vi "DAQmx Create Channel (TEDS-AI-Force-IEPE Sensor).vi"(0 "task in":refnum<k21>, 1 "maximum value":dbl=2000.0 format="%0.2f", 2 "minimum value":dbl=-2000.0 format="%0.2f", 3 "input terminal configuration":i32(ring)=-1 items=["default"=-1, "RSE"=10083, "NRSE"=10078, "Differential"=10106, "Pseudodifferential"=12529], 5 "physical channels":tag, 6 "current excitation source":i32(ring)=10200 items=["Internal"=10200, "External"=10167, "None"=10230], 7 "name to assign":string, 8 "current excitation value":dbl=0.001, 9 "units":i32(ring)=15875 items=["Newtons"=15875, "Pounds"=15876, "From Custom Scale"=10065], 11 "error in":errorcluster, 12 "custom scale name":tag) -> (4 "task out":refnum<k21>, 15 "error out":errorcluster)   [LabVIEW 2018]
doc: "Creates channel(s) that use an IEPE force sensor to measure force or load. You must configure the physical channel(s) with TEDS information to use this VI."
uses:
  nilvaiu.dll
panel:
  # "input limits"
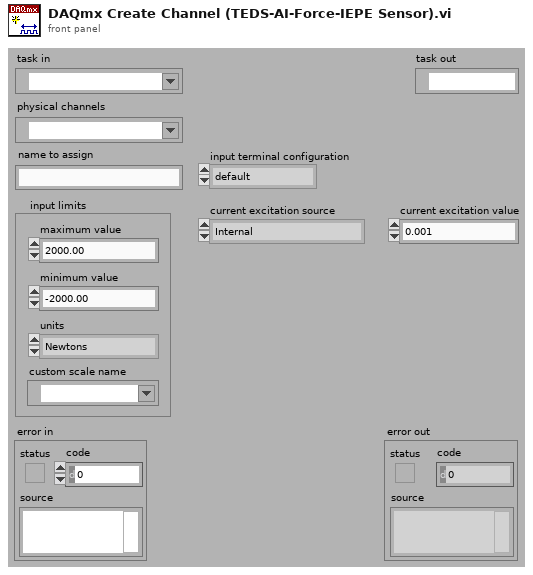
[diagram p1: front panel]
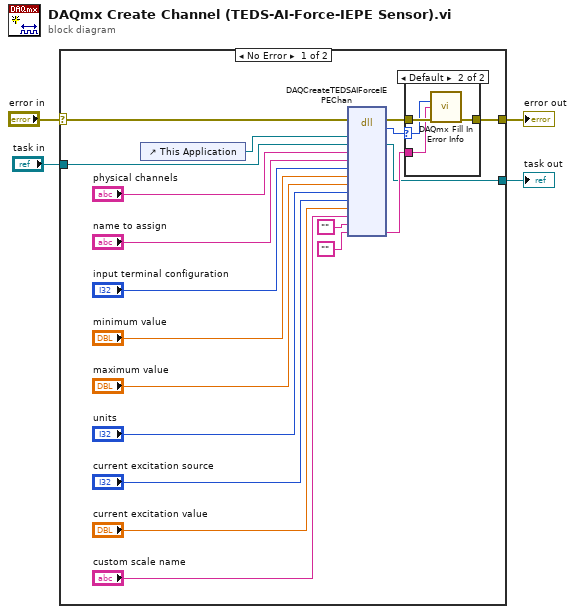
[diagram p0: block diagram]
diagram:
  n1 = case shown="No Error" "error in" {
    selector: "error in" -> [w18 w30]
    tunnel: [w17 w30] -> w2
    tunnel: "task in" -> [w16 w29]
    tunnel: [w15 w29] -> w1
    frame No Error {
      n2 = control-ref of="This Application"() -> (w20:refnum<vi>)
      n3 = dll-call lib="nilvaiu.*" fn="DAQCreateTEDSAIForceIEPEChan"(error in=w18, "lvAppRef"=w20, "refObjPtr"=w16, "physicalChannelName"="physical channels", "channelNameIn"="name to assign", "terminalConfig"="input terminal configuration", "minVal"="minimum value", "maxVal"="maximum value", "units"="units", "currentExcitSrc"="current excitation source", "excitVal"="current excitation value", "customScaleName"="custom scale name", "channelNamesOut"="", "extendedErrorInfo"="") -> (error out=w23:errorcluster, "return type"=w22:i32, "refObjPtr"=w15:refnum<k21>, "extendedErrorInfo"=w21:string)  [unwired: 13 in, 1 out]
      n4 = case shown="Default" w22 {
        selector: w22 -> [_ w26]
        tunnel: w23 -> [w24 w28]
        tunnel: [w24 w27] -> w17
        tunnel: w21 -> [_ w25]
        frame 0 {
        }
        frame Default {
          n5 = call "DAQmx Fill In Error Info.vi"("status code"=w26, "extended error info"=w25, "error in"=w28) -> ("error out"=w27:errorcluster)  [unwired: 1 in, 11 out]
        }
      }
    }
    frame Error {
    }
  }
  "error out" <- w2
  "task out" <- w1
